vi "example_areOverlapped.vi"() -> ()   [LabVIEW 2023]
uses:
  TLC_Scripto.lvlib
  BlockDiagram/BlockDiagram.lvclass
  Terminal/Terminal.lvclass
panel:
  out "areObjectsOverlapped?":bool
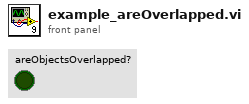
[diagram p1: front panel]
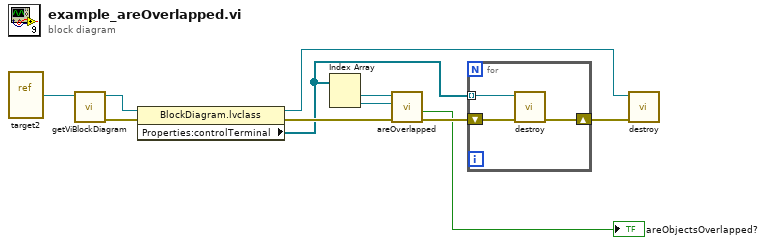
[diagram p0: block diagram]
diagram:
  n1 = vi-ref "target2.vi"() -> (w11:refnum<vi>)
  n2 = call "getViBlockDiagram.vi"("ViRef"=w11) -> ("error out"=w10:errorcluster, "topMostBlockDiagram"=w9:refnum<class "BlockDiagram.lvclass">)  [unwired: 9 in]
  n3 = property class="BlockDiagram.lvclass"(reference=w9, error in=w10) -> (reference out=w7:refnum<class "BlockDiagram.lvclass">, error out=w4:errorcluster, "Properties:controlTerminal"=w2:refnum<class "Terminal.lvclass">[])
  n4 = Index Array(array=w2) -> (element #1=w6:refnum<class "Terminal.lvclass">, element #2=w5:refnum<class "Terminal.lvclass">)  [unwired: 2 in]
  n5 = call "areOverlapped.vi"("error in (no error)"=w4, "GObject2"=w5, "GObject1"=w6) -> ("error out"=w3:errorcluster, "areObjectsOverlapped?"=→"areObjectsOverlapped?":bool)  [unwired: 5 in, 2 out]
  n6 = for {
    shift-right: [w14] -> w8
    shift-left: w3 -> [w13]
    tunnel: w2 -> [w12] mode=indexing
    n7 = call-dynamic "destroy.vi"("Error In"=w13, "Generic In"=w12) -> ("Error Out"=w14:errorcluster)  [unwired: 9 in]
  }
  n8 = call-dynamic "destroy.vi"("Error In"=w8, "Generic In"=w7) -> ()  [unwired: 9 in, 1 out]
